vi "Get Engine Offset.vi"(11 "Transfer Configuration in":refnum<class "Transfer Configuration.lvclass">) -> (2 "engine offset":u64, 3 "Transfer Configuration out":refnum<class "Transfer Configuration.lvclass">)   [LabVIEW 2017, in "DSF Core.lvlib" / "Transfer Configuration.lvclass"]
uses:
  Transfer Configuration.lvclass
  Transfer Configuration.lvclass/Transfer Configuration.ctl
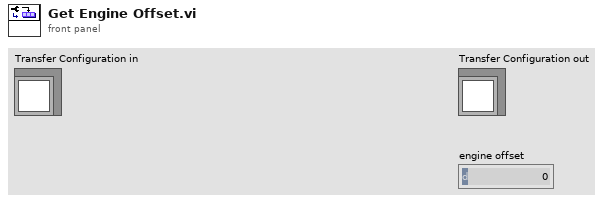
[diagram p1: front panel]
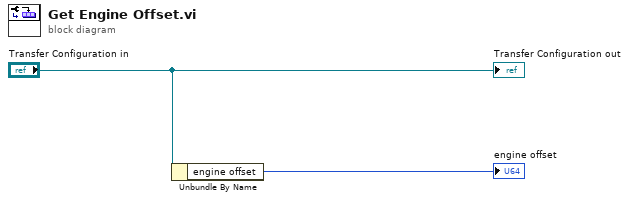
[diagram p0: block diagram]
diagram:
  n1 = Unbundle By Name("Transfer Configuration in") -> ("engine offset"=→"engine offset":u64)
  "Transfer Configuration out" <- "Transfer Configuration in"
